vi "Return Weight Precheck.vi"(8 "error in":errorcluster, 10 "Weight Number":i32, 11 "GrabberTool in":refnum<class "GrabberTool Class.lvclass">) -> (0 "error out":errorcluster, 3 "GrabberTool out":refnum<class "GrabberTool Class.lvclass">)   [LabVIEW 2011, in "GrabberTool Class.lvclass"]
uses:
  GrabberTool Class.lvclass
  GrabberTool Class.lvclass/GrabberTool Class.ctl
  WorkTable Class/WorkTable Class.lvclass
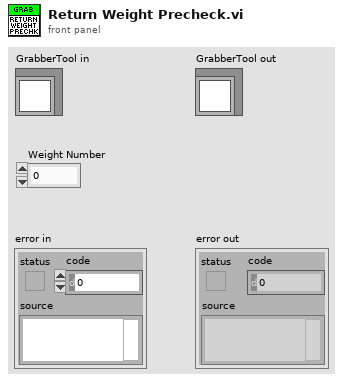
[diagram p1: front panel]
types:
  T1 = typedef "Worktable_Weights.ctl" = cluster{"Weight Slots":cluster{"Weight State":enum16{"Empty", "Populated"}, "Weight Type":T2, "Location/Orientation":T3}[], "Vacuum Channel":i32}
  T2 = typedef "Weight Type.ctl" = enum16{"Weight 1", "Weight 2", "Weight 3", "Weight 4", "Weight 5", "Weight 6", "Weight 7", "Weight 8"}
  T3 = typedef "Position_Orientation.ctl" = cluster{"Center":refnum<class "Vec3d Class.lvclass">, "Orientation":refnum<class "Orient3d Class.lvclass">}
  T4 = cluster{"Weight State":enum16{"Empty", "Populated"}, "Weight Type":T2, "Location/Orientation":T3}[]
  T5 = cluster{"Weight State":enum16{"Empty", "Populated"}, "Weight Type":T2, "Location/Orientation":T3}
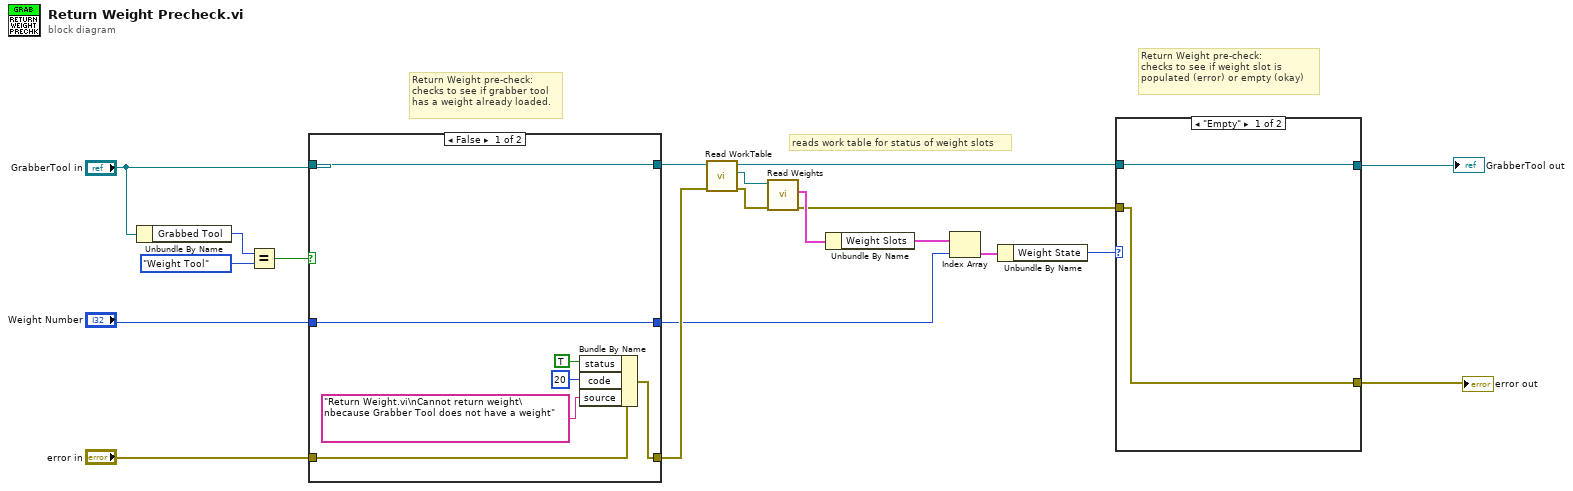
[diagram p0: block diagram]
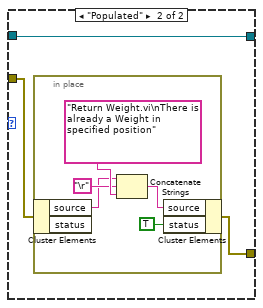
[diagram p2: hidden frame]
diagram:
  # "Return Weight pre-check:\nchecks to see if weight slot is\npopulated (error) or empty (okay)"
  # "reads work table for status of weight slots"
  # "Return Weight pre-check:\nchecks to see if grabber tool\nhas a weight already loaded."
  n1 = Unbundle By Name("GrabberTool in") -> ("Grabbed Tool"=w18:enum16{"Weight Tool", "Stamp Tool", "Nothing"})
  n2 = Equal?(x=w18, y=enum16{"Weight Tool", "Stamp Tool", "Nothing"}."Weight Tool") -> (x = y?=w4:bool)
  n3 = case shown="False" w4 {
    tunnel: [w26 w29] -> w16
    tunnel: "GrabberTool in" -> [w26 w29]
    tunnel: [w20 w27] -> w15
    tunnel: "error in" -> [w21 w27]
    tunnel: [w25 w28] -> w10
    tunnel: "Weight Number" -> [w25 w28]
    frame False {
      n4 = Bundle By Name(cluster=w21, "status"=TRUE, "code"=20, "source"="Return Weight.vi\nCannot return weight\nbecause Grabber Tool does not have a weight") -> (w20:errorcluster)
    }
    frame True {
    }
  }
  n5 = call-dynamic "Read WorkTable.vi"("error in"=w15, "Gantry Class in"=w16) -> ("error out"=w13:errorcluster, "WorkTable Class.lvclass"=w14:refnum<class "WorkTable Class.lvclass">, "Gantry Class out"=w7:refnum<class "GrabberTool Class.lvclass">)  [unwired: 7 in]
  n6 = call-dynamic "Read Weights.vi"("error in (no error)"=w13, "WorkTable Class in"=w14) -> ("error out"=w6:errorcluster, "Weights"=w12:T1)  [unwired: 7 in, 1 out]
  n7 = Unbundle By Name(w12) -> ("Weight Slots"=w11:T4)
  n8 = Index Array(array=w11, index=w10) -> (element=w9:T5)
  n9 = Unbundle By Name(w9) -> ("Weight State"=w8:enum16{"Empty", "Populated"})
  n10 = case shown="\"Empty\"" w8 {
    tunnel: w7 -> [w31 w34]
    tunnel: [w31 w34] -> w1
    tunnel: w6 -> [w30 w32]
    tunnel: [w30 w33] -> w2
    frame "Empty" {
    }
    frame "Populated" {
      n11 = in-place {
        n12 = in-place-cluster #1(w32) -> ("source"=w36:string)  [unwired: 1 out]
        n13 = Concatenate Strings(w36, "\r", "Return Weight.vi\nThere is already a Weight in specified position" ("string")) -> (w37:string)
        n14 = in-place-cluster #1("source"=w37, "status"=TRUE) -> (w33:errorcluster)
      }
    }
  }
  "error out" <- w2
  "GrabberTool out" <- w1
